vi "PID tester line follower.vi"   [LabVIEW 2016]
types:
  T1 = typedef "LVHSConnector.ctl" = refnum<class "BrickReference.lvclass">
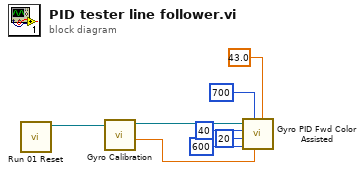
[diagram p0: block diagram]
diagram:
  n1 = call "Run 01 Reset.vi"() -> ("NXT/EV3 out"=w6:T1)  [unwired: 11 in]
  n2 = call "Gyro Calibration.vi"("NXT/EV3"=w6) -> ("Degrees"=w1:sgl, "NXT/EV3"=w7:T1)  [unwired: 6 in, 1 out]
  n3 = call "Gyro PID Fwd Color Assisted.vi"("Target reflection"=sgl 43.0, "Target angle"=w1, "Threshold to Color"=700 ("Threshold to stop"), "Threshold to slow"=600, "Min. speed"=20, "Max. speed"=40, "EV3 in"=w7) -> ()  [unwired: 4 in, 1 out]
